vi "07 - Benchmark - Effect of Number of Subscribers on Event Post Time.vi"() -> ()   [LabVIEW 2012]
panel:
  out "Benchmark":cluster{i32[], u32[]}(graph) caption="This graph demonstrates that the amount of time to post a message scales linearly\nwith the number of subscribers to that messenger."
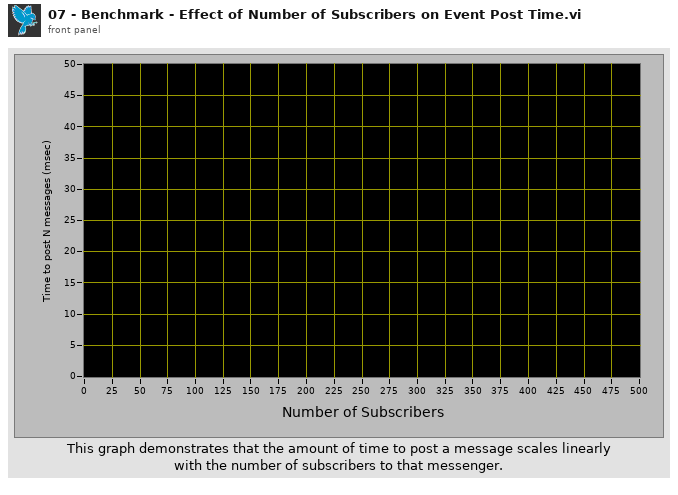
[diagram p1: front panel]
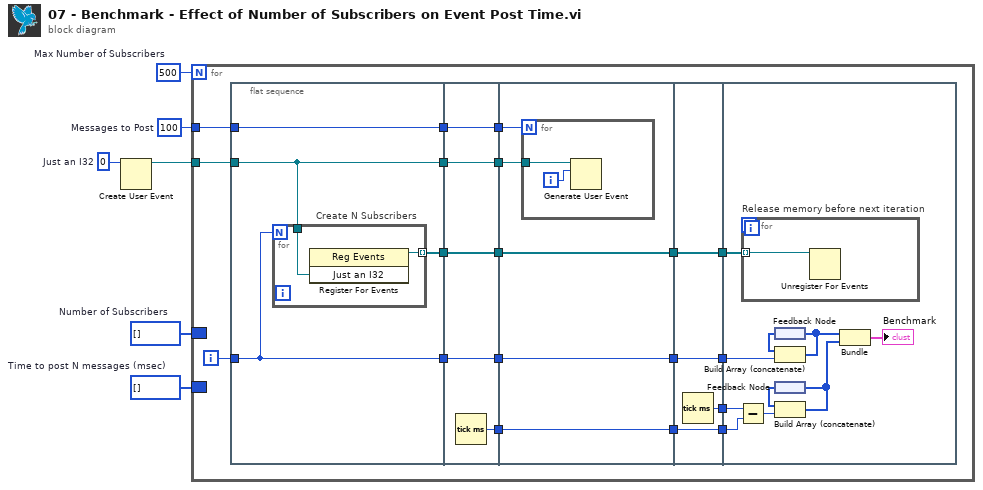
[diagram p0: block diagram]
diagram:
  w1 = i32[] []  # Number of Subscribers
  w2 = u32[] []  # Time to post N messages (msec)
  w5 = 500  # Max Number of Subscribers
  w3 = 100  # Messages to Post
  w6 = 0  # Just an I32
  n1 = Create User Event(user event datatype=w6) -> (user event=w4:refnum<user-event>)  [unwired: 1 in, 1 out]
  n2 = for {
    N: w5 -> [_]
    tunnel: w4 -> [w13]
    tunnel: w3 -> [w12]
    border: w2 -> [_]
    border: w1 -> [_]
    i -> [w11]
    n3 = flat-sequence {
      tunnel: [w27] -> w25
      tunnel: [w28] -> w24
      tunnel: [w29] -> w23
      tunnel: [w26] -> w7
      tunnel: w11 -> [w26]
      tunnel: w12 -> [w27]
      tunnel: w13 -> [w28]
      tunnel: [w36] -> w22
      tunnel: w25 -> [w36]
      tunnel: [w35] -> w21
      tunnel: w24 -> [w35]
      tunnel: w23 -> [w34]
      tunnel: [w34] -> w20
      tunnel: [w33] -> w19
      tunnel: [w32] -> w8
      tunnel: w7 -> [w32]
      tunnel: w22 -> [w40]
      tunnel: w21 -> [w41]
      tunnel: [w39] -> w18
      tunnel: w20 -> [w39]
      tunnel: [w38] -> w17
      tunnel: w19 -> [w38]
      tunnel: [w37] -> w9
      tunnel: w8 -> [w37]
      tunnel: [w47] -> w16
      tunnel: w18 -> [w47]
      tunnel: [w46] -> w15
      tunnel: [w45] -> w14
      tunnel: w17 -> [w45]
      tunnel: [w44] -> w10
      tunnel: w9 -> [w44]
      tunnel: w16 -> [w57]
      tunnel: w15 -> [w56]
      tunnel: w14 -> [w53]
      tunnel: w10 -> [w54]
      frame #0 {
        n4 = for "Create N Subscribers" {
          N: w26 -> [_]
          tunnel: [w31] -> w29 mode=indexing
          tunnel: w28 -> [w30]
          n5 = register-events(w30) -> (reference out=w31:refnum<event-registration>)  [unwired: 2 in, 1 out]
        }
      }
      frame #1 {
        n6 = Tick Count (ms)() -> (millisecond timer value=w33:u32)
      }
      frame #2 {
        n7 = for {
          N: w40 -> [_]
          tunnel: w41 -> [w43]
          i -> [w42]
          n8 = Generate User Event(user event=w43, event data cluster=w42) -> ()  [unwired: 1 in, 2 out]
        }
      }
      frame #3 {
        n9 = Tick Count (ms)() -> (millisecond timer value=w46:u32)
      }
      frame #4 {
        n10 = Subtract(x=w56, y=w53) -> (x-y=w55:u32)
        n11 = for "Release memory before next iteration" {
          tunnel: w57 -> [w58] mode=indexing
          n12 = Unregister For Events(event registration refnum=w58) -> ()  [unwired: 1 in, 1 out]
        }
        n13 = feedback #1() -> (w50:i32[])
        n14 = Build Array (concatenate)(w50, w54) -> (w51:i32[])
        n15 = feedback-in #1(w51) -> ()
        n16 = feedback #2() -> (w49:u32[])
        n17 = Build Array (concatenate)(w49, w55) -> (w48:u32[])
        n18 = feedback-in #2(w48) -> ()
        n19 = Bundle(w51, w48) -> (→"Benchmark":cluster{i32[], u32[]})  [unwired: 1 in]
      }
    }
  }
